vi "EyeBlinkConditioning_extinction.vi"() -> ()   [LabVIEW 2013]
uses:
  <vilib>/Platform/TimedLoop/XDataNode/timing_clust.ctl
  <vilib>/Platform/TimedLoop/XDataNode/nitl_modes.ctl
  <vilib>/Platform/TimedLoop/XDataNode/wakeup.ctl
  <vilib>/Utility/file.llb/Write To Spreadsheet File (string).vi
  <vilib>/platform/TimedLoop/XDataNode/XDataNode.xnode
  <vilib>/Platform/TimedLoop/XDataNode/XDNodeRunTimeDep.lvlib
panel:
  out "CS (Tone)":bool
  out "next trial":string
  out "CS Trial indexs & time":string[][](array[string])
  out "US (Air Puff)":bool
  out "Total trial/session":i32
  in  "Mouse ID":string="N2#07"
  in  "file path (dialog if empty)":path=path "C:/Users/George Augustine Lab/Helen-treadmill/pmr-Helen/EyeBlinkConditioning/EyeBlink_Data/20211113/20211113_EyeBlink_extinction_N2#07"
  out "current trial duration (ms)":dbl
  in  "stop task":bool
  out "Task Duration (min)":dbl
  out "No. of Trials":dbl
  out "ITI (s) [next-current]":dbl
  # "Extinction"
  # "#100 US only trials \n#100 CS only trials\n#US only trials and CS only trials are alternatively deliveried\n#ITI is randomly between 10s and 20s"
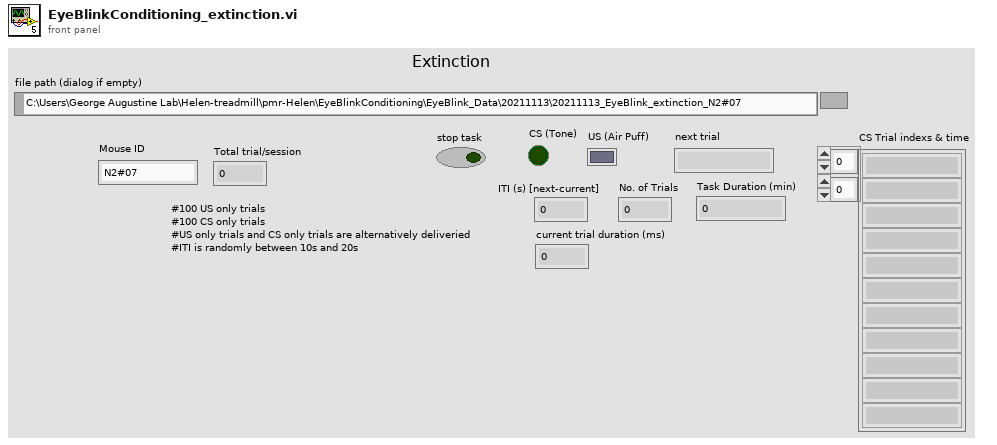
[diagram p1: front panel]
types:
  T1 = typedef "XDNodeRunTimeDep.lvlib/timing_clust.ctl" = cluster{"Expected End [f-1]":u64, "Actual End [f-1]":u64, "Finished Late? [f-1]":bool, "Expected End [i-1]":u64, "Actual End [i-1]":u64, "Finished Late? [i-1]":bool, "Expected Start [i]":u64, "Actual Start [i]":u64, "Expected Start [f]":u64, "Actual Start [f]":u64, "Source Name":string, "Structure Name":string, "Period":i64, "Deadline":i64, "Offset":i64, "Start":i64, "Priority":i32, "Timeout":i32, "Mode":T2, "Wakeup Reason":T3, "Error":errorcluster, "Source Type":string, "Secondary Source Type":string, "Global End Time":u64, "Global Start Time":u64, "Frame Duration":u64, "Iteration Duration":u64, "Assigned CPU":i32, "I/O Scan Engine Mode":u32}
  T2 = typedef "XDNodeRunTimeDep.lvlib/nitl_modes.ctl" = enum32{"No Change", "Process missed periods, maintain original phase", "Discard missed periods, maintain original phase", "Process missed periods, ignore original phase", "Discard missed periods, ignore original phase"}
  T3 = typedef "XDNodeRunTimeDep.lvlib/wakeup.ctl" = enum32{"Normal", "Aborted", "Asynchronous wakeup", "Timing source error", "Timed loop error", "Timeout"}
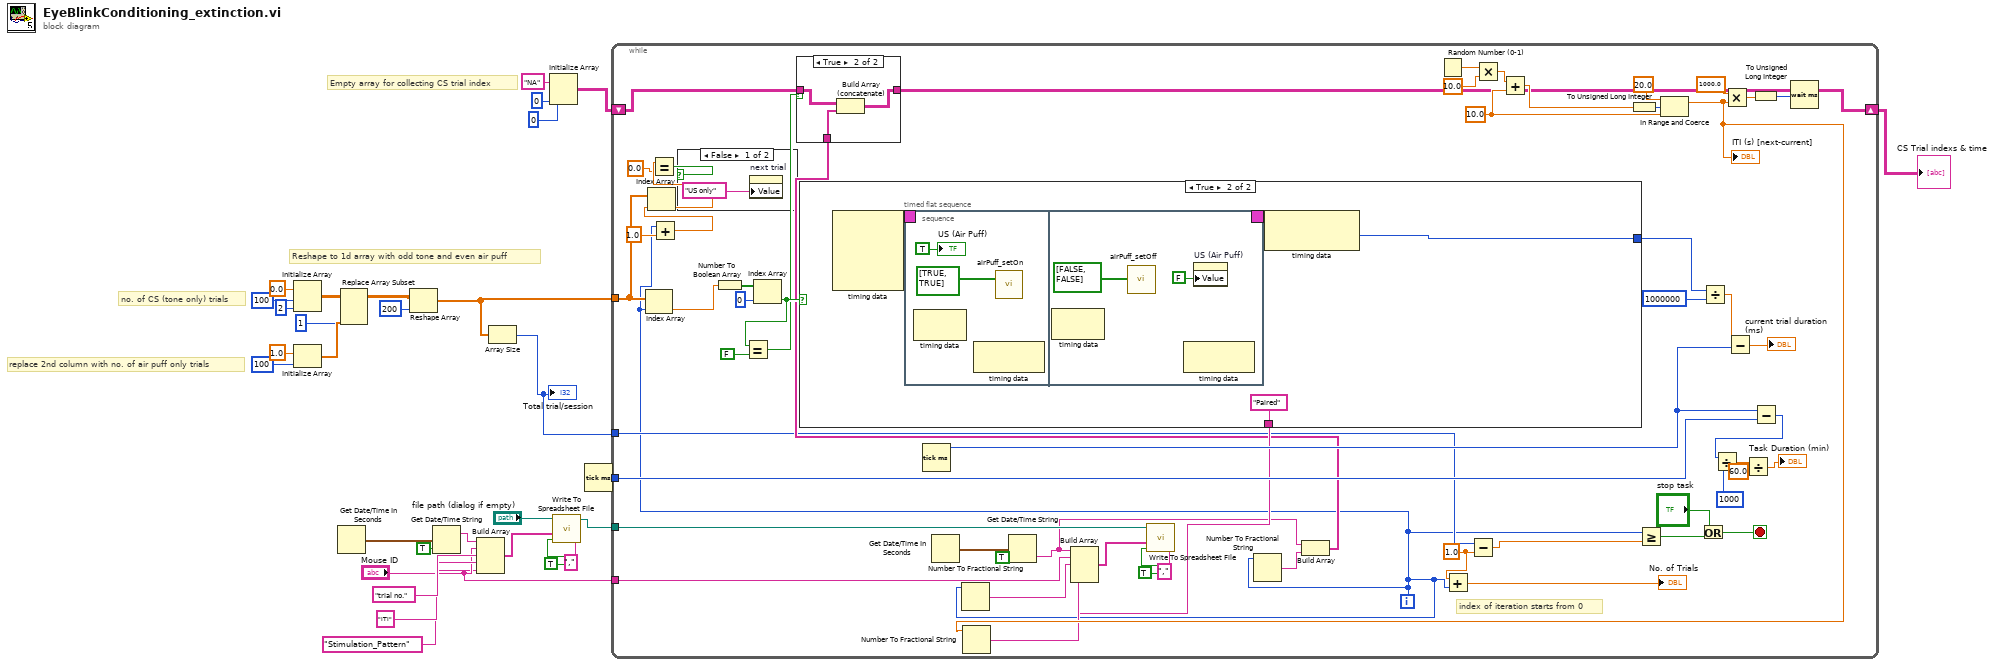
[diagram p0: block diagram]
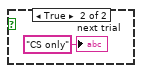
[diagram p2: hidden frame]
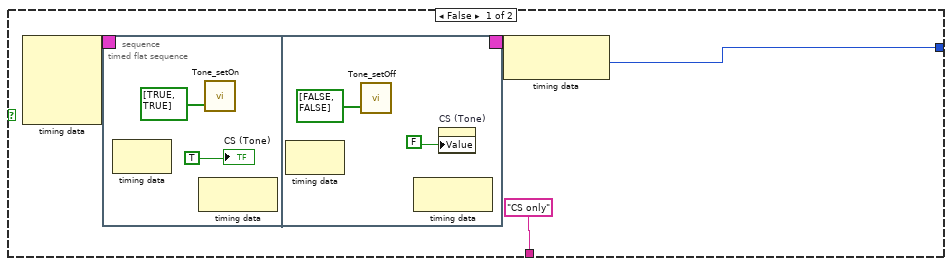
[diagram p4: hidden frame]
diagram:
  # "Reshape to 1d array with odd tone and even air puff"
  # "Empty array for collecting CS trial index"
  # "replace 2nd column with no. of air puff only trials"
  # "no. of CS (tone only) trials"
  n1 = Initialize Array(0.0 ("element"), 100 ("dimension size"), 2 ("dimension size")) -> (w5:dbl[][])
  n2 = Initialize Array(1.0 ("element"), 100 ("dimension size")) -> (w9:dbl[])
  n3 = Get Date/Time In Seconds() -> (seconds since 1Jan1904=w25:timestamp)
  n4 = Replace Array Subset(array=w5, new element=w9, index (col)=1 ("disabled index (col)")) -> (w10:dbl[][])  [unwired: 1 in]
  n5 = Reshape Array(w10, 200 ("dimension size")) -> (w1:dbl[])
  n6 = Get Date/Time String(seconds (now)=w25, want seconds? (F)=TRUE) -> (date string=w24:string)  [unwired: 1 in, 1 out]
  n7 = Build Array(w24, "Mouse ID", "trial no." ("element"), "ITI" ("element"), "Stimulation_Pattern" ("element")) -> (w21:string[])
  n8 = Array Size(array=w1) -> (size(s)=w18:i32)
  "Total trial/session" <- w18
  n9 = Initialize Array("NA" ("element"), 0 ("dimension size"), 0 ("dimension size")) -> (w13:string[][])
  n10 = call-poly <vilib>:"Write To Spreadsheet File.vi"("delimiter (\\t)"="," ("delimiter (\\t)"), "append to file? (new file:F)"=TRUE, "1D data"=w21, "file path (dialog if empty)"="file path (dialog if empty)") -> ("new file path (Not A Path if cancelled)"=w20:path)  [unwired: 4 in]
  n11 = Tick Count (ms)() -> (millisecond timer value=w30:u32)
  n12 = while {
    tunnel: w30 -> [w71]
    tunnel: w20 -> [w62]
    tunnel: "Mouse ID" -> [w61]
    tunnel: w1 -> [w41]
    tunnel: w18 -> [w35]
    shift-right: [w45] -> w12
    shift-left: w13 -> [w50]
    i -> [w31]
    stop <- w77 stop-if-true
    w33 = 1.0 ("y")
    w85 = 10.0 ("Randomized ITI between (s)")
    # "index of iteration starts from 0"
    n13 = Index Array(array=w41, index=w31) -> (element=w54:dbl)
    n14 = Add(x=w31, y=1.0) -> (x+y=w39:dbl)
    n15 = Index Array(array=w41, index=w39) -> (element=w37:dbl)
    n16 = Equal?(x=w37, y=0.0) -> (x = y?=w38:bool)
    n17 = case shown="False" w38 {
      frame False {
        n18 = property on="next trial" class="Str"("Value"="US only" ("next trial")) -> ()  [unwired: 2 in, 2 out]
      }
      frame True {
        "next trial" <- "CS only" ("next trial")
      }
    }
    n19 = Number To Boolean Array(number=w54) -> (Boolean array=w56:bool[])
    n20 = Index Array(array=w56, index=0) -> (element=w52:bool)
    n21 = Equal?(x=w52, y=FALSE) -> (x = y?=w49:bool)
    n22 = case shown="True" w52 {
      tunnel: [w95 w110] -> w57
      tunnel: ["CS only" "Paired"] -> w53
      frame False {
        n23 = node-c288() -> (w97:T1)  [unwired: 4 in]
        n24 = timed-sequence {
          timing: w97 -> [_]
          timing-out: [_] -> w96
          n25 = timed-flat-sequence {
            frame #0 {
              n26 = node-c288() -> ()  [unwired: 1 in, 1 out]
              n27 = node-c288() -> ()  [unwired: 1 in, 1 out]
              n28 = call "Tone_setOn"("data"=bool[] [TRUE, TRUE]) -> ()  [unwired: 17 in, 2 out]
              "CS (Tone)" <- TRUE ("CS (LED)")
            }
            frame #1 {
              n29 = node-c288() -> ()  [unwired: 1 in, 1 out]
              n30 = call "Tone_setOff"("data"=bool[] [FALSE, FALSE]) -> ()  [unwired: 17 in, 2 out]
              n31 = node-c288() -> ()  [unwired: 1 in, 1 out]
              n32 = property on="CS (Tone)" class="Bool (strict)"("Value"=FALSE ("CS (LED)")) -> ()  [unwired: 2 in, 2 out]
            }
          }
        }
        n33 = node-c288(w96) -> (w95:i64)
      }
      frame True {
        n34 = node-c288() -> (w112:T1)  [unwired: 4 in]
        n35 = timed-sequence {
          timing: w112 -> [_]
          timing-out: [_] -> w111
          n36 = timed-flat-sequence {
            frame #0 {
              n37 = node-c288() -> ()  [unwired: 1 in, 1 out]
              n38 = node-c288() -> ()  [unwired: 1 in, 1 out]
              n39 = call "airPuff_setOn"("data"=bool[] [TRUE, TRUE]) -> ()  [unwired: 17 in, 2 out]
              "US (Air Puff)" <- TRUE ("US (Air Puff)")
            }
            frame #1 {
              n40 = node-c288() -> ()  [unwired: 1 in, 1 out]
              n41 = call "airPuff_setOff"("data"=bool[] [FALSE, FALSE]) -> ()  [unwired: 17 in, 2 out]
              n42 = node-c288() -> ()  [unwired: 1 in, 1 out]
              n43 = property on="US (Air Puff)" class="Bool (strict)"("Value"=FALSE ("US (Air Puff)")) -> ()  [unwired: 2 in, 2 out]
            }
          }
        }
        n44 = node-c288(w111) -> (w110:i64)
      }
    }
    n45 = Tick Count (ms)() -> (millisecond timer value=w70:u32)
    n46 = Get Date/Time In Seconds() -> (seconds since 1Jan1904=w66:timestamp)
    n47 = Number To Fractional String(number=w31) -> (F-format string=w58:string)  [unwired: 3 in]
    n48 = Get Date/Time String(seconds (now)=w66, want seconds? (F)=TRUE) -> (time string=w47:string)  [unwired: 1 in, 1 out]
    n49 = Number To Fractional String(number=w31) -> (F-format string=w48:string)  [unwired: 3 in]
    n50 = Build Array(w47, w48) -> (w46:string[])
    n51 = case shown="True" w49 {
      tunnel: w50 -> [w90 w93]
      tunnel: w46 -> [_ w92]
      tunnel: [w90 w91] -> w45
      frame False {
      }
      frame True {
        n52 = Build Array (concatenate)(w93, w92) -> (w91:string[][])
      }
    }
    n53 = Random Number (0-1)() -> (number: 0 to 1=w83:dbl)
    n54 = Add(x=w33, y=w31) -> (x+y=→"No. of Trials":dbl)
    n55 = Subtract(x=w35, y=w33) -> (x-y=w34:dbl)
    n56 = Multiply(x=w83, y=10.0) -> (x*y=w84:dbl)
    n57 = Add(x=w84, y=w85) -> (x+y=w86:dbl)
    n58 = To Unsigned Long Integer(number=w86) -> (unsigned 32bit integer=w82:u32)
    n59 = Greater Or Equal?(x=w31, y=w34) -> (x >= y?=w76:bool)
    n60 = In Range and Coerce(upper limit=20.0 ("And (s)"), x=w82, lower limit=w85) -> (coerced(x)=w60:dbl)  [unwired: 1 out]
    "ITI (s) [next-current]" <- w60
    n61 = Number To Fractional String(number=w60) -> (F-format string=w59:string)  [unwired: 3 in]
    n62 = Build Array(w47, w61, w58, w59, w53) -> (w67:string[])
    n63 = call-poly <vilib>:"Write To Spreadsheet File.vi"("delimiter (\\t)"="," ("delimiter (\\t)"), "append to file? (new file:F)"=TRUE, "1D data"=w67, "file path (dialog if empty)"=w62) -> ()  [unwired: 4 in, 1 out]
    n64 = Or(x="stop task", y=w76) -> (x .or. y?=w77:bool)
    n65 = Divide(x=w57, y=i64 1000000) -> (x/y=w68:dbl)
    n66 = Multiply(x=1000.0, y=w60) -> (x*y=w79:dbl)
    n67 = Subtract(x=w68, y=w70) -> (x-y=→"current trial duration (ms)":dbl)
    n68 = To Unsigned Long Integer(number=w79) -> (unsigned 32bit integer=w78:u32)
    n69 = Subtract(x=w70, y=w71) -> (x-y=w73:u32)
    n70 = Divide(x=w73, y=u32 1000) -> (x/y=w44:dbl)
    n71 = Divide(x=w44, y=60.0) -> (x/y=→"Task Duration (min)":dbl)
    n72 = Wait (ms)(milliseconds to wait=w78) -> ()  [unwired: 1 out]
  }
  "CS Trial indexs & time" <- w12
